vi "main.vi"() -> ()   [LabVIEW 2019]
uses:
  CodeModule/gui/RUNNING.ctl
  CodeModule/gui/LeSSeN.ctl
  CodeModule/gui/add.ctl
  CodeModule/core/core_reportMode.ctl
  CodeModule/core/core_reportCfg.ctl
  CodeModule/gui/ps_setting.ctl
  CodeModule/gui/LIMIT DATA.ctl
  CodeModule/instrument/Instrument.lvclass
  CodeModule/core/core_dataCluster.ctl
panel:
  out "日期/时间":string
  in  "Save data":bool
  in  "Settings":bool
  out "Torque":T1
  out "ECU":T1
  out "Load":T1
  out "DC Power":T1
  out "ECU SATE":i16
  out "System EFF":dbl format="%#_4f"
  out "ECU EFF":dbl format="%#_4f"
  out "Motor":dbl format="%#_5f"
  out "Motor EFF":dbl format="%#_4f"
  out "Motor Power":dbl format="%#_4g"
  out "Pha Power":dbl format="%#_6f"
  out "Pha Current":dbl format="%#_4f"
  out "Pha V":dbl format="%#_4f"
  out "DC Power":dbl format="%#_4f"
  out "Toque":dbl format="%#_4f"
  out "Motor":dbl format="%#_4g"
  out "Drive":dbl format="%#_4f"
  out "Logic V":dbl format="%#_4g"
  out "Temp 2":dbl format="%#_4f"
  out "Temp 1":dbl format="%#_4f"
  out "Speed":dbl format="%#_5f"
  out "Torque":dbl format="%#_4f"
  out "DCCurrent":dbl format="%#_5f"
  out "DC V":dbl format="%#_4f"
  in  "ECU ACK":bool
  in  "load mode":enum32{"torque", "spedd"}(tab)
  in  "Set LoadDivide":dbl(slide) min=0.0 max=2000.0 scale=0.0..5000.0
  in  "Load NM -":T2
  in  "LoadNM+":T3
  out "Load Divide":dbl(knob) scale=1.0..5000.0 scale format="%#_4g"
  in  "StepDivide":dbl
  in  "LOAD ACK Nm":bool
  in  "LOAD ACK":bool
  in  "设定Load[rpm]":i32(slide) min=0 max=4000 step=1 scale=0.0..4000.0
  in  "rpm -":T2
  in  "rpm +":T3
  out "r/m":dbl(knob) scale=0.0..4000.0 scale format="%#.4g"
  in  "Step rpm":i32
  in  "Step Torque":dbl
  out "Troque N/m":dbl(knob) scale=0.0..200.0 scale format="%#_4g"
  in  "Nm -":T2
  in  "Nm +":T3
  in  "Set Torque[Nm]":sgl(slide) min=0 max=200 step=0.1 scale=0.0..200.0
  in  "load direction":bool
  in  "finish":bool
  out "State":string
  out "Finish Time":timestamp format="%<%H:%M:%S\n%x>T"
  out "Start Time":timestamp format="%<%H:%M:%S\n%x>T"
  in  "report cfg":T4
  in  "Duration [min]":i32=30
  in  "Data Mode":T5
  in  "Report File Path":path
  in  "Profile File Path":path
  in  "Cycle Time":i32=1
  out "DATA":string[][](table)
  in  "load torque":bool
  out "CYC  Times":dbl format="%#_7g"
  out "Run Time":dbl format="%<%H:%M:%S>t"
  in  "load 2":bool
  in  "ecu":bool
  in  "ps":bool
  in  "zlg":bool
  in  "play":bool
  in  "emergency stop":bool
  # "BST-1500-22KW电力测功机系统"
  # "MOTOR"
  # "rpm"
  # "N/m"
  # "KW"
  # "DC Power"
  # "V"
  # "A"
  # "KW"
  # "ZLG"
  # "KW"
  # "V"
  # "A"
  # "%"
  # "%"
  # "%"
  # "ECU"
  # "V"
  # "℃"
  # "℃"
  # "ECU"
  # "rpm"
  # "℃"
  # "Temp"
  # "℃"
  # "℃"
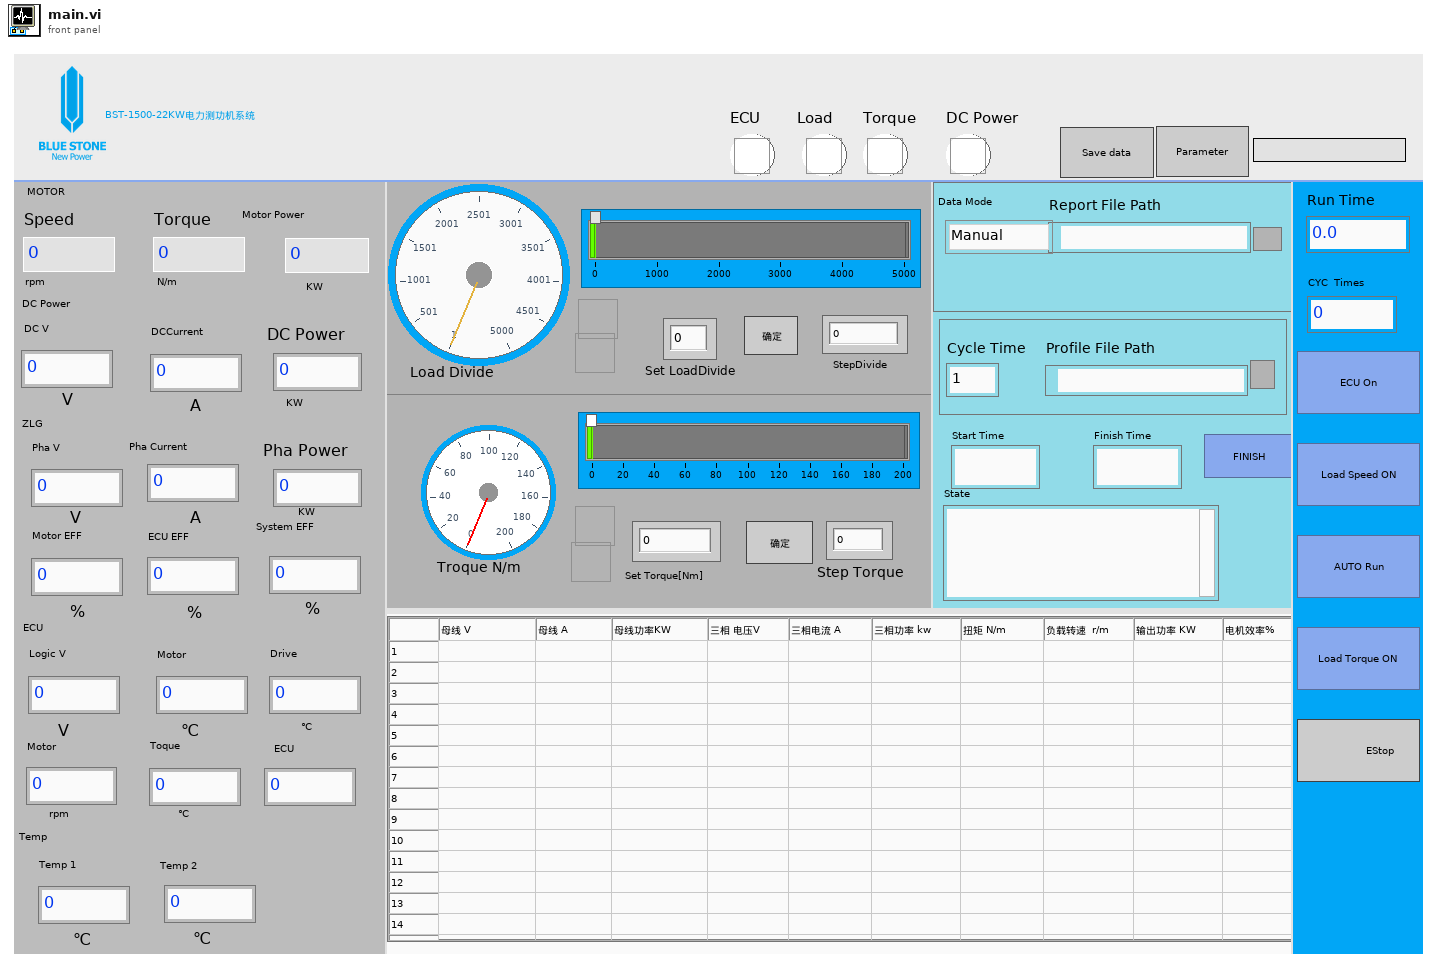
[diagram p1: front panel]
types:
  T1 = typedef "RUNNING.ctl" = bool
  T2 = typedef "LeSSeN.ctl" = bool
  T3 = typedef "add.ctl" = bool
  T4 = typedef "core_reportCfg.ctl" = cluster{"Path":path, "duration(min)":i32, "mode":T5}
  T5 = typedef "core_reportMode.ctl" = enum16{"Manual", "Automatic"}
  T6 = typedef "LIMIT DATA.ctl" = cluster{"Motor Temp Limit ":dbl, " Motor Speed Limit ":dbl, "AXIS Temp Limit  ":dbl, " Torque Limit":dbl, " Speed   limt":dbl}
  T7 = typedef "ps_setting.ctl" = cluster{"母线电压":sgl, "母线电流":sgl, "过载电压":sgl, "过载电流":sgl}
  T8 = typedef "select.ctl" = bool
  T9 = cluster{"Error event ref out":refnum<user-event>, "ecuData":refnum<user-event>}
  T10 = typedef "core_dataRefCluster.ctl" = cluster{"modbus":T11, "ecu":T11, "test":T11}
  T11 = typedef "core_dataRef.ctl" = refnum<queue>
  T12 = typedef "core_dataCluster.ctl" = cluster{"cmd":string, "data":variant}
  T13 = cluster{"母线电压":sgl, "母线电流":sgl, "过载电压":sgl, "过载电流":sgl, "ps":bool}
  T14 = typedef "core_setup.ctl" = cluster{"time":i32, "torque":dbl, "speed":i32}
  T15 = typedef "profile value.ctl" = cluster{"time in":i32, "speed":dbl, "Torque":dbl}
  T16 = typedef "Instrument.lvclass/instr_dataCluster.ctl" = cluster{"电源电压 V":dbl, "电源电流A":dbl, "扭矩N/m":dbl, "速度r/M":dbl, "温度℃":dbl[], "流量计L/M":dbl[]}
  T17 = typedef "core shown data.ctl" = cluster{"SHOWN":dbl[], "temp 2":dbl, "ECU EFF":dbl, "SYS EFF":dbl, "temp 1":dbl}
  T18 = enum8{"Enabled", "Disabled", "Disabled and Grayed Out"}
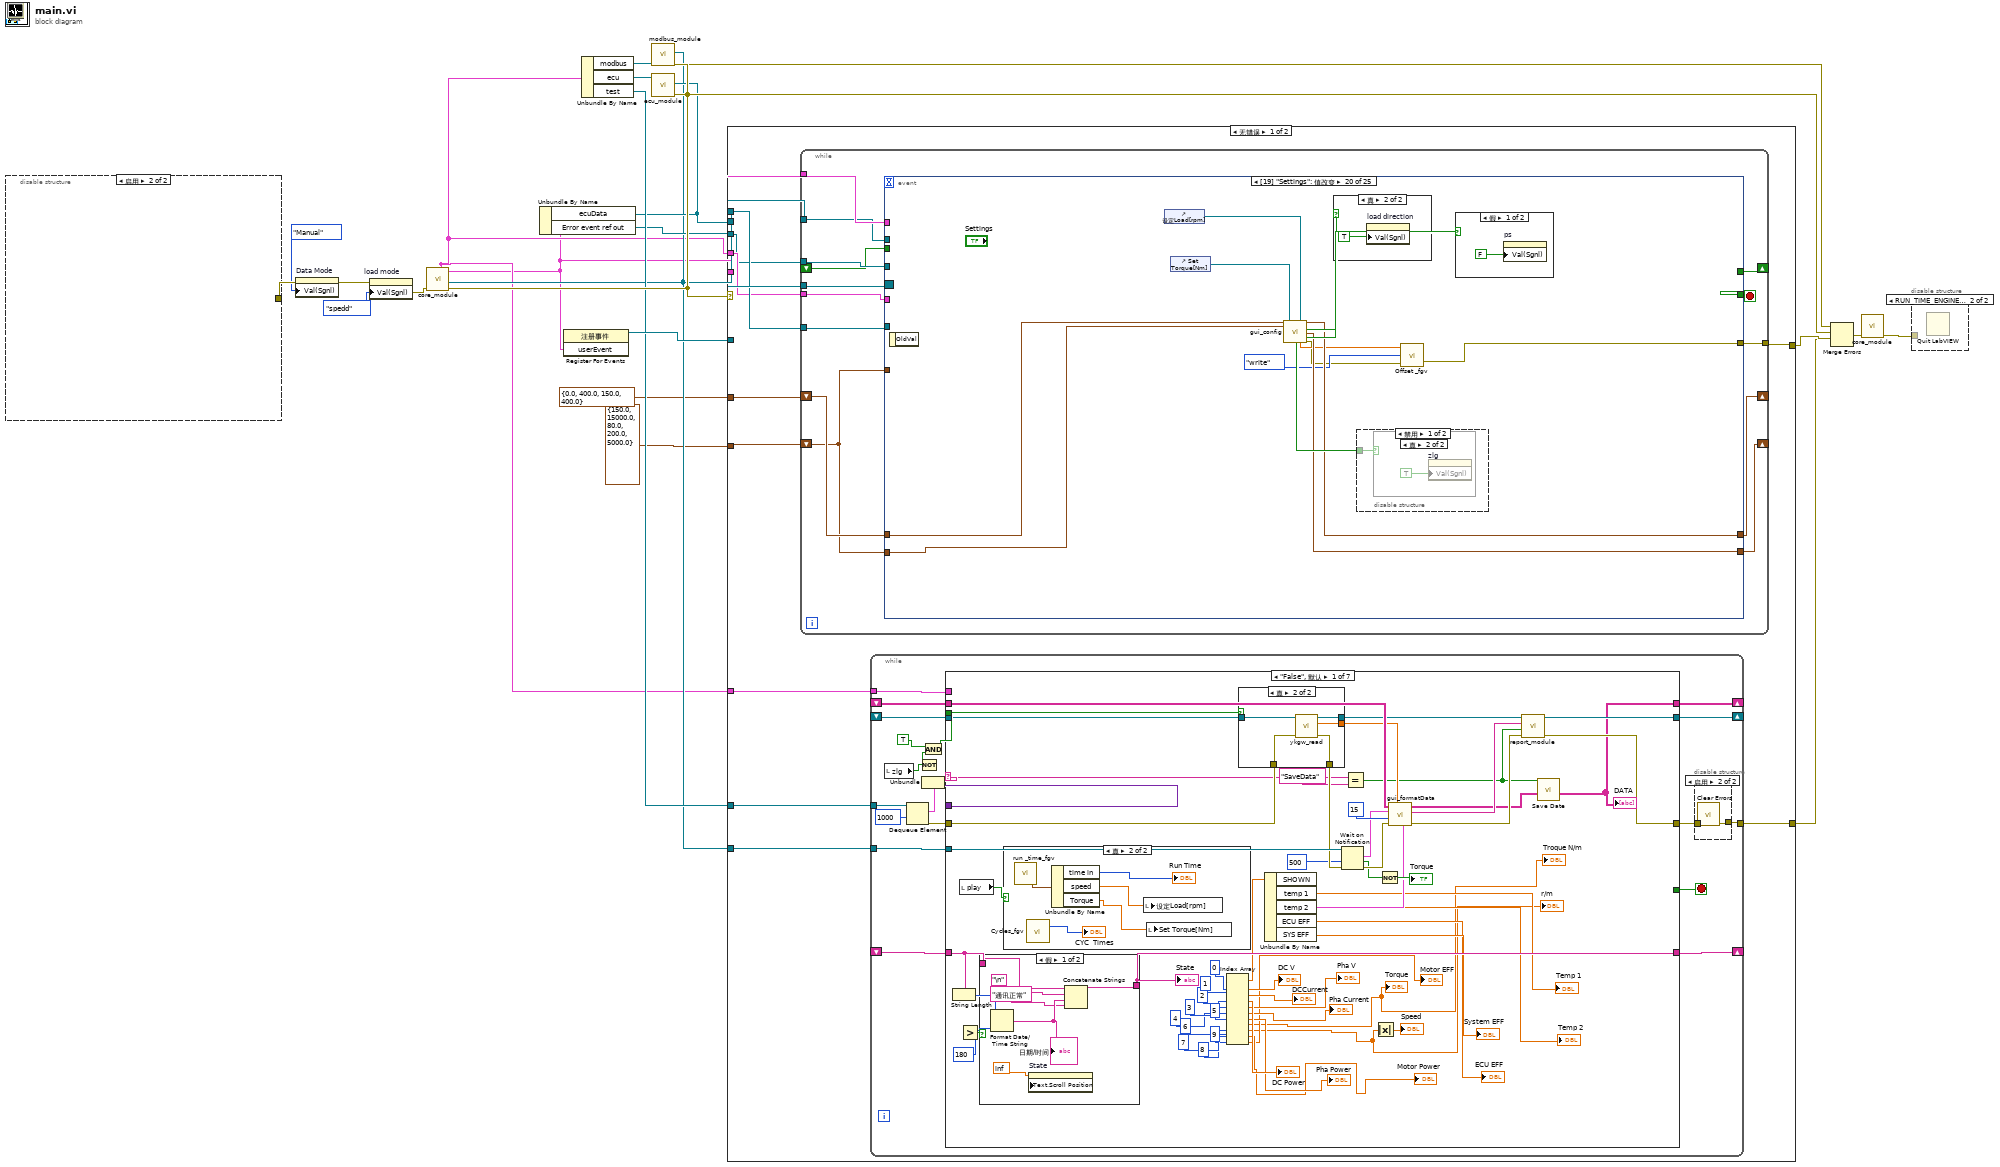
[diagram p0: block diagram]
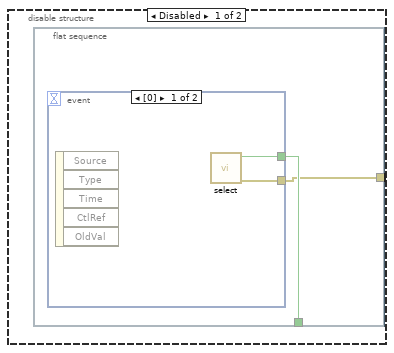
[diagram p2: hidden frame]
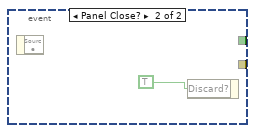
[diagram p3: hidden frame]
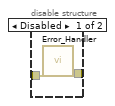
[diagram p4: hidden frame]
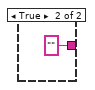
[diagram p5: hidden frame]
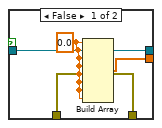
[diagram p6: hidden frame]
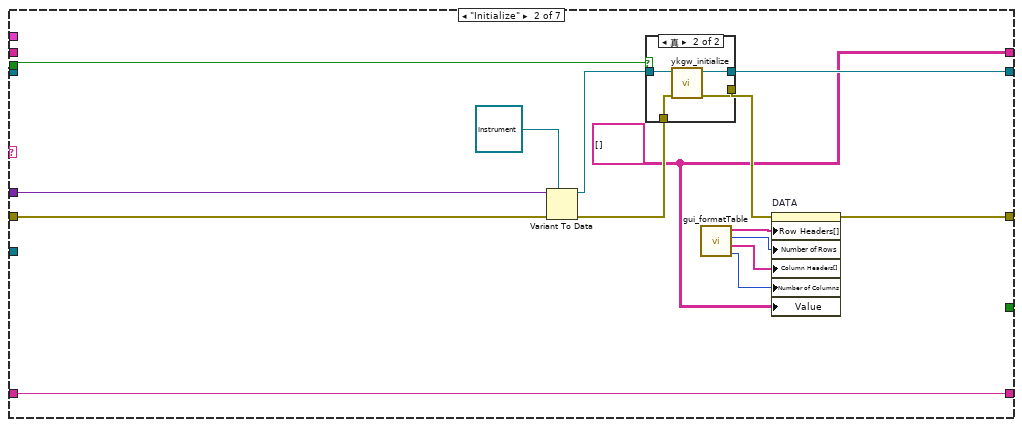
[diagram p8: hidden frame]
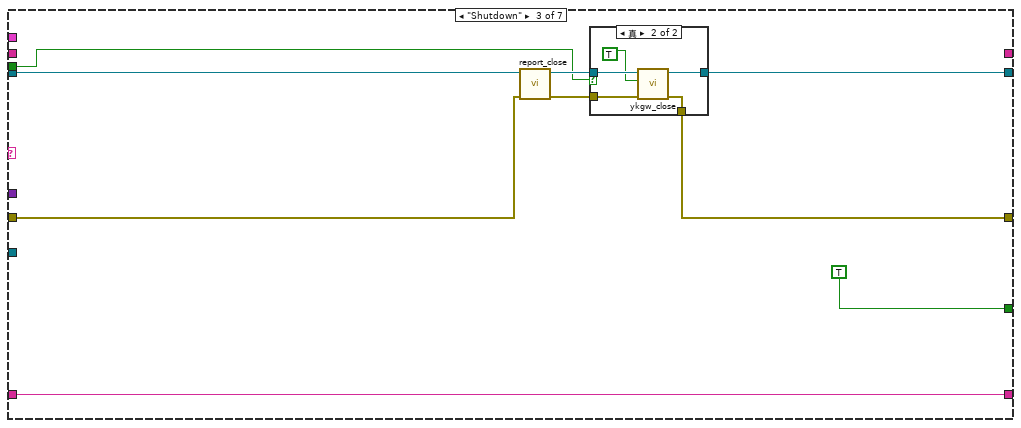
[diagram p10: hidden frame]
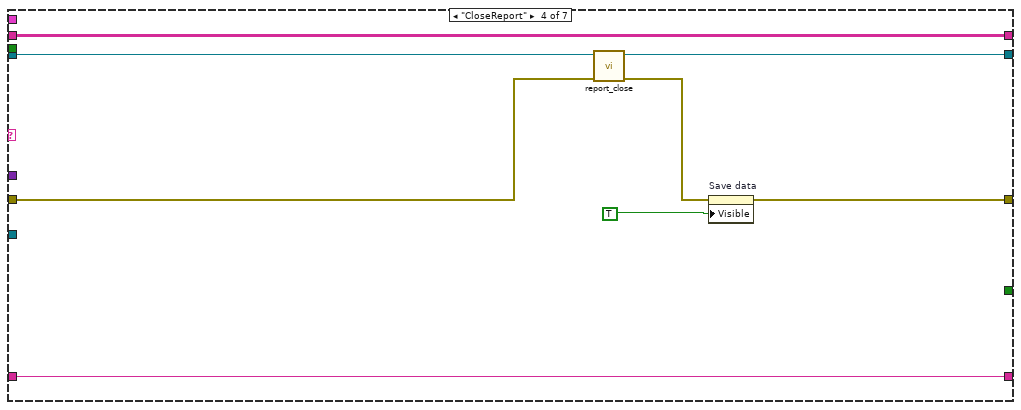
[diagram p12: hidden frame]
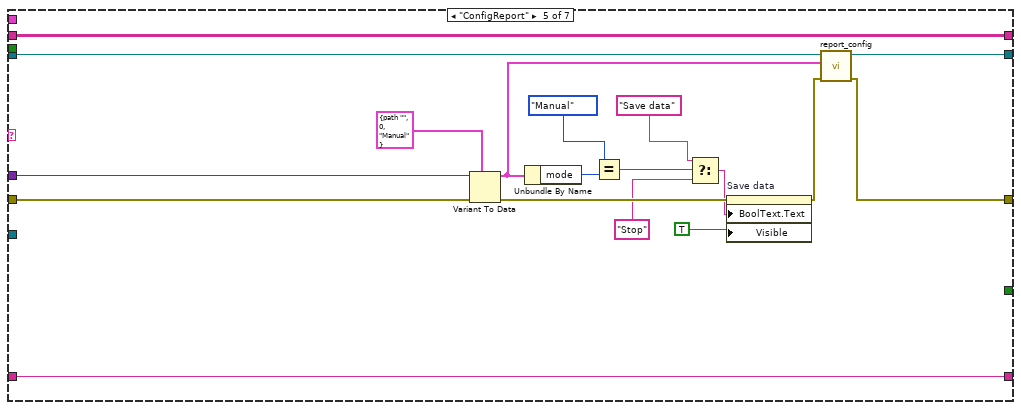
[diagram p13: hidden frame]
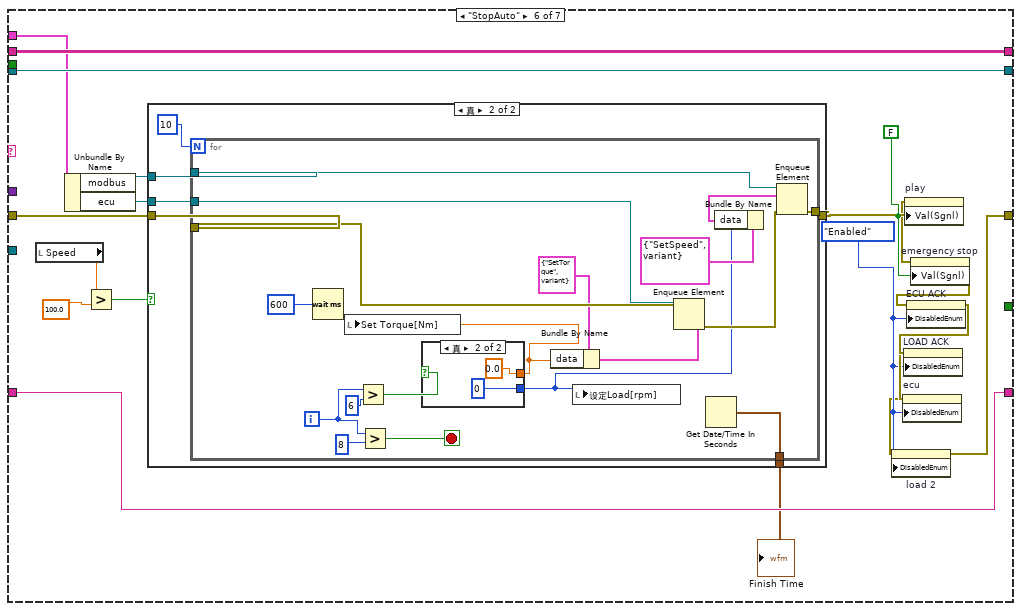
[diagram p14: hidden frame]
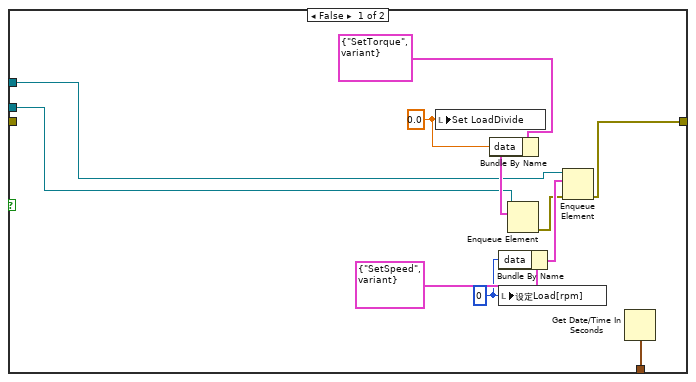
[diagram p15: hidden frame]
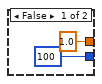
[diagram p16: hidden frame]
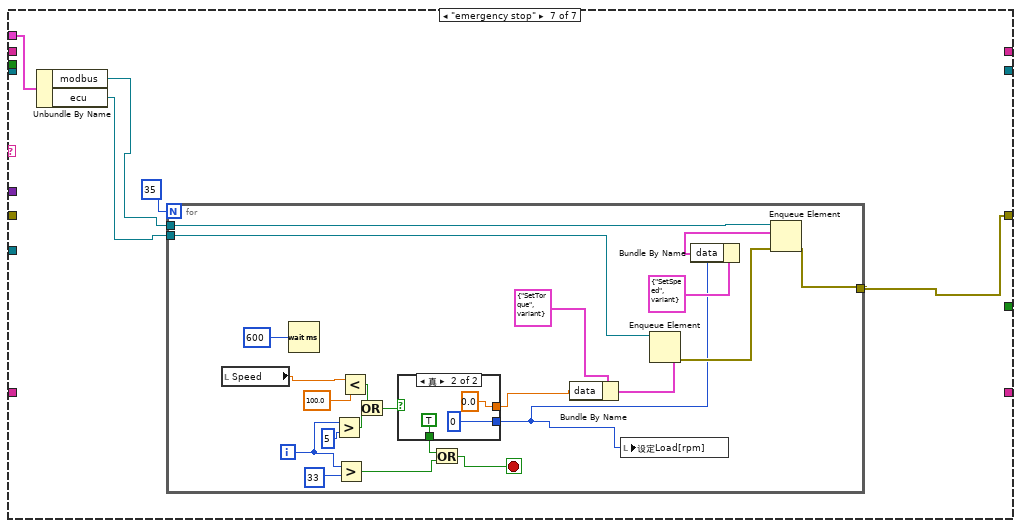
[diagram p17: hidden frame]
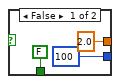
[diagram p18: hidden frame]
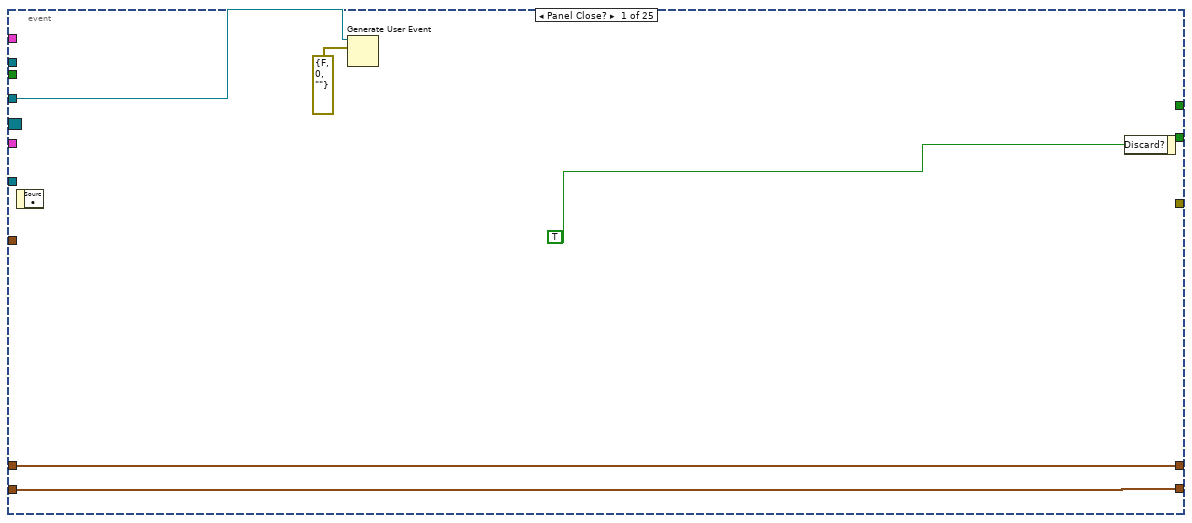
[diagram p19: hidden frame]
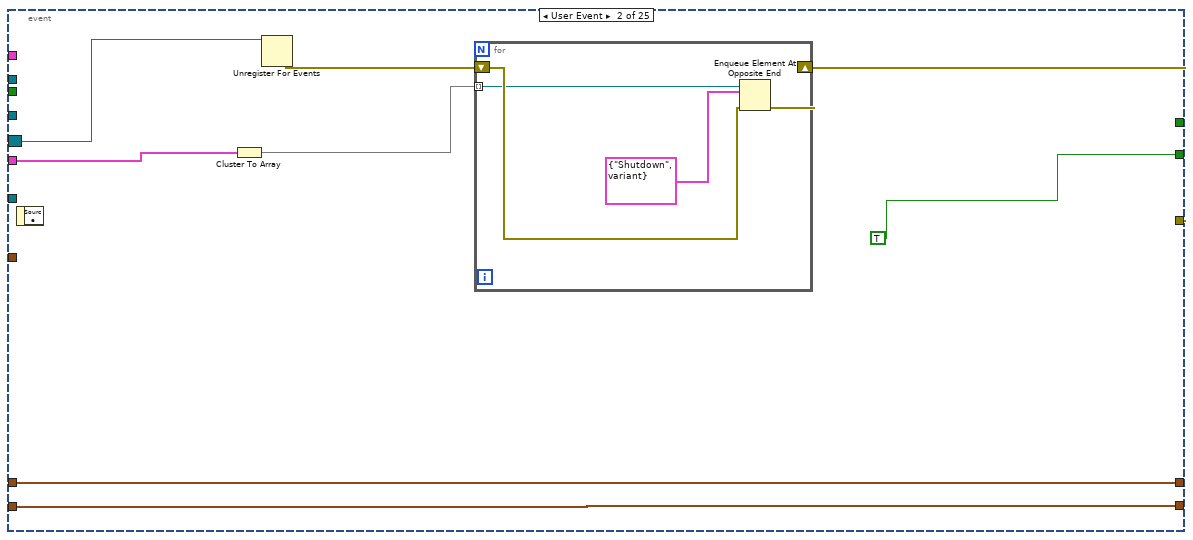
[diagram p20: hidden frame]
diagram:
  n1 = disable-structure shown="启用" {
    disable-tunnel: [w24 _] -> w5
    frame Disabled {
      n2 = flat-sequence {
        tunnel: [w26] -> _
        tunnel: [w25] -> w24
        frame #0 {
          n3 = event shown="[0]" {
            selector: _ -> [_ _]
            dyn-events: _ -> [_ _]
            timeout: _ -> [_ _]
            tunnel: [w28 _] -> w25
            tunnel: [w27 _] -> w26
            event #0 (no event record) {
              n4 = event-data() -> ()  [unwired: 1 in, 5 out]
              n5 = call "select.vi"() -> ("out"=w27:T8, "error out"=w28:errorcluster)  [unwired: 9 in]
            }
            event Panel Close? {
              n6 = event-data() -> ()  [unwired: 1 in, 1 out]
              n7 = event-data("Discard?"=TRUE) -> ()  [unwired: 1 in, 1 out]
            }
          }
        }
      }
    }
    frame Enabled {
    }
  }
  n8 = property on="Data Mode" class="Enum (严格)"(error in=w5, "Val(Sgnl)"=core_reportMode."Manual" ("值(信号)")) -> (error out=w3:errorcluster)  [unwired: 1 in, 1 out]
  n9 = property on="load mode" class="TabCtl (严格)"(error in=w3, "Val(Sgnl)"=enum32{"torque", "spedd"}."spedd" ("load mode")) -> (error out=w1:errorcluster)  [unwired: 1 in, 1 out]
  n10 = call "core_module.vi"("error in (no error)"=w1) -> ("error out"=w19:errorcluster, "modbusData"=w11:refnum<notifier>, "userEvent"=w6:T9, "Cluster"=w9:T10)  [unwired: 6 in, 1 out]
  n11 = Unbundle By Name(w6) -> ("ecuData"=w12:refnum<user-event>, "Error event ref out"=w13:refnum<user-event>)
  n12 = register-events(w6) -> (reference out=w23:refnum<event-registration>)  [unwired: 2 in, 1 out]
  n13 = Unbundle By Name(w9) -> ("modbus"=w16:T11, "ecu"=w15:T11, "test"=w14:T11)
  n14 = call "modbus_module.vi"("error in (no error)"=w19, "User Event"=w11, "queue in"=w16) -> ("error out"=w18:errorcluster)  [unwired: 8 in]
  n15 = call "ecu_module.vi"("error in (no error)"=w19, "ecuData"=w12, "queue in"=w15) -> ("error out"=w20:errorcluster)  [unwired: 8 in]
  n16 = case shown="无错误" w19 {
    tunnel: w6 -> [w42 _]
    tunnel: w23 -> [w41 _]
    tunnel: w9 -> [w31 _]
    tunnel: [w33 _] -> w22
    tunnel: w14 -> [w40 _]
    tunnel: [w39 _] -> w17
    tunnel: w11 -> [w38 _]
    tunnel: w13 -> [w30 _]
    tunnel: w12 -> [w37 _]
    tunnel: w11 -> [w32 _]
    tunnel: T7 {"母线电压"=0.0, "母线电流"=400.0, "过载电压"=150.0, "过载电流"=400.0} ("PS Setting") -> [w34 _]
    tunnel: w9 -> [w36 _]
    tunnel: T6 {"Motor Temp Limit "=150.0, " Motor Speed Limit "=15000.0, "AXIS Temp Limit  "=80.0, " Torque Limit"=200.0, " Speed   limt"=5000.0} ("LIMIT") -> [w35 _]
    frame No Error {
      n17 = while {
        tunnel: w42 -> [w313]
        tunnel: w41 -> [w312]
        tunnel: w30 -> [w311]
        tunnel: w37 -> [w310]
        tunnel: w32 -> [w309]
        shift-right: [w305] -> _
        shift-left: _ -> [w308]
        shift-right: [w302] -> _
        shift-left: w35 -> [w300]
        shift-right: [w303] -> _
        shift-left: w34 -> [w307]
        tunnel: [w304] -> w33
        tunnel: w31 -> [w301]
        stop <- w306 stop-if-true
        n18 = event shown="[19] \"Settings\": 值改变" {
          selector: w312 -> [_ w326 _ _ _ _ _ _ _ _ _ _ _ _ _ _ _ _ _ _ _ _ _ _ _]
          dyn-events: _ -> [_ _ _ _ _ _ _ _ _ _ _ _ _ _ _ _ _ _ _ _ _ _ _ _ _]
          timeout: _ -> [_ _ _ _ _ _ _ _ _ _ _ _ _ _ _ _ _ _ _ _ _ _ _ _ _]
          tunnel: w313 -> [_ _ _ _ _ _ _ _ _ _ _ _ _ _ _ _ _ _ _ _ _ _ _ _ _]
          tunnel: w301 -> [_ w324 _ w378 w394 w415 w423 w428 w446 w477 w491 w508 w531 w542 w557 w580 w596 w607 w612 _ w671 w699 w708 _ w764]
          tunnel: [_ w322 w344 w379 w393 w401 w417 w429 w441 w472 w492 w509 w529 w540 w556 w574 w586 w605 w617 w629 w666 w698 w707 w751 w758] -> w304
          tunnel: w311 -> [w317 _ _ _ _ _ _ _ _ _ _ _ _ _ _ _ _ _ _ _ _ _ _ _ _]
          tunnel: w310 -> [_ _ _ _ _ _ _ _ _ _ _ _ _ _ _ _ _ _ _ _ _ _ _ _ _]
          tunnel: w309 -> [_ _ w361 _ _ _ _ _ _ _ _ _ _ _ _ _ _ _ _ _ _ _ _ _ _]
          tunnel: w308 -> [_ _ w360 _ w390 _ _ _ _ _ _ _ _ _ _ _ _ _ _ _ _ _ _ _ _]
          tunnel: w300 -> [_ _ w343 _ _ _ _ _ _ _ _ _ _ _ _ _ _ _ _ _ _ _ _ _ _]
          tunnel: w300 -> [w314 w319 w340 w375 w389 w402 w416 w424 w440 w461 w487 w503 w524 w536 w553 w575 w585 w600 w616 w634 w656 w683 w704 w749 w754]
          tunnel: w307 -> [w316 w320 w342 w376 w391 w403 w418 w425 w442 w462 w488 w504 w525 w537 w554 w576 w587 w601 w621 w635 w657 w684 w705 w750 w755]
          tunnel: [w314 w319 w340 w375 w389 w402 w416 w424 w440 w461 w487 w503 w524 w536 w553 w575 w585 w600 w616 w632 w656 w683 w704 w749 w754] -> w302
          tunnel: [_ TRUE _ _ _ _ _ _ _ _ _ _ _ _ _ _ _ _ _ _ _ _ _ _ _] -> w306
          tunnel: [_ _ w341 _ w390 _ _ _ _ _ _ _ _ _ _ _ _ _ w615 _ _ _ _ _ _] -> w305
          tunnel: [w316 w320 w342 w376 w391 w403 w418 w425 w442 w462 w488 w504 w525 w537 w554 w576 w587 w601 w621 w633 w657 w684 w705 w750 w755] -> w303
          event Panel Close? {
            n19 = event-data() -> ()  [unwired: 1 in, 1 out]
            n20 = Generate User Event(user event=w317, event data cluster=errorcluster {"status"=FALSE, "code"=0, "source"=""} ("event data")) -> ()  [unwired: 2 in, 2 out]
            n21 = event-data("Discard?"=TRUE) -> ()  [unwired: 1 in, 1 out]
          }
          event User Event {
            n22 = event-data() -> ()  [unwired: 1 in, 1 out]
            n23 = Cluster To Array(cluster=w324) -> (array=w323:T11[])
            n24 = Unregister For Events(event registration refnum=w326) -> (error out=w325:errorcluster)  [unwired: 1 in]
            n25 = for {
              tunnel: w323 -> [w327] mode=indexing
              shift-right: [w328] -> w322
              shift-left: w325 -> [w330]
              n26 = Enqueue Element At Opposite End(queue=w327, element=T12 {"cmd"="Shutdown", "data"=variant}, error in (no error)=w330) -> (error out=w328:errorcluster)  [unwired: 1 in, 2 out]
            }
          }
          event User Event {
            n27 = event-data() -> ("MCU_MotTq"=→"Toque":dbl, "MCU_MotBusU"=→"Logic V":dbl, "MCU_MotSpd"=w331:dbl, "MCU_MotCtrlrT"=→"Drive":dbl, "MCU_MotBodyT"=→"Motor":dbl, "MCU 状态"=w336:bool)  [unwired: 1 in, 2 out]
            "Motor" <- w331
            n28 = Unbundle By Name(w343) -> ("Motor Temp Limit"=w354:dbl, "Motor Speed Limit"=w339:dbl, "AXIS Temp Limit"=w359:dbl, "Torque Limit"=w352:dbl, "Speed   limt"=w351:dbl)
            n29 = local read "Temp 1"() -> (w358:dbl)
            n30 = local read "Torque"() -> (w347:dbl)
            n31 = local read "Speed"() -> (w345:dbl)
            n32 = local read "Motor"() -> (w355:dbl)
            n33 = Greater?(x=w331, y=w339) -> (0:w338:bool)
            n34 = Greater?(x=w358, y=w359) -> (0:w348:bool)
            n35 = Greater?(x=w345, y=w351) -> (0:w350:bool)
            n36 = Absolute Value(x=w347) -> (abs(x)=w346:dbl)
            n37 = Greater?(x=w355, y=w354) -> (0:w356:bool)
            n38 = Greater?(x=w346, y=w352) -> (0:w353:bool)
            n39 = Compound Arithmetic op=OR ("复合运算")(w353, w356, w350, w348, w338) -> (w349:bool)
            n40 = Boolean To (0,1)(Boolean=w336) -> (0, 1=→"ECU SATE":i16)
            n41 = case shown="假" w349 {
              tunnel: [FALSE TRUE] -> w337
              frame False {
              }
              frame True {
              }
            }
            n42 = disable-structure shown="启用" {
              disable-tunnel: w361 -> [w367 _]
              disable-tunnel: w360 -> [w365 _]
              disable-tunnel: [w364 _] -> w344
              disable-tunnel: [w363 _] -> w341
              frame Disabled {
                n43 = call "gui_checkEmergencyStop.vi"("Check"=w365, "modbusData"=w367) -> ("error out"=w366:errorcluster, "Stop"=w362:bool, "Continue check"=w363:bool)  [unwired: 7 in]
                n44 = case shown="真" w362 {
                  tunnel: w366 -> [w368 w372]
                  tunnel: w362 -> [_ w371]
                  tunnel: [w368 w370] -> w364
                  frame False {
                  }
                  frame True {
                    n45 = Not(x=w371) -> (.not. x?=w369:bool)
                    n46 = property on="emergency stop" class="Bool (严格)"(error in=w372, "Val(Sgnl)"=w369) -> (error out=w370:errorcluster)  [unwired: 1 in, 1 out]
                  }
                }
              }
              frame Enabled {
              }
            }
            n47 = property on="emergency stop" class="Bool (严格)"("Val(Sgnl)"=w337) -> ()  [unwired: 2 in, 2 out]
          }
          event "ps": Value Change {
            n48 = event-data() -> ()  [unwired: 1 in, 1 out]
            n49 = Unbundle By Name(w376) -> ("母线电压"=w386:sgl, "母线电流"=w385:sgl, "过载电压"=w384:sgl, "过载电流"=w383:sgl)
            n50 = Bundle(cluster=T13 {"母线电压"=0.0, "母线电流"=0.0, "过载电压"=0.0, "过载电流"=0.0, "ps"=FALSE} ("簇"), "母线电压"=w386, "母线电流"=w385, "过载电压"=w384, "过载电流"=w383, "ps"="ps") -> (w381:T13)
            n51 = Bundle By Name(cluster=T12 {"cmd"="PS", "data"=variant} ("element"), "data"=w381) -> (w387:T12)
            n52 = Unbundle By Name(w378) -> ("modbus"=w377:T11)
            n53 = Enqueue Element(queue=w377, element=w387) -> (error out=w379:errorcluster)  [unwired: 2 in, 2 out]
            "DC Power" <- "ps"
          }
          event "zlg": Value Change {
            n54 = event-data() -> ("NewVal"=w392:bool)  [unwired: 1 in]
            n55 = disable-structure shown="禁用" {
              disable-tunnel: w394 -> [w400 _]
              disable-tunnel: [w398 _] -> w393
              disable-tunnel: w392 -> [w395 _]
              frame Disabled {
                n56 = Unbundle By Name(w400) -> ("modbus"=w399:T11)
                n57 = Bundle By Name(cluster=T12 {"cmd"="EnableChiller", "data"=variant} ("element"), "data"=w395) -> (w396:T12)
                n58 = Enqueue Element(queue=w399, element=w396) -> (error out=w398:errorcluster)  [unwired: 2 in, 2 out]
              }
              frame Enabled {
              }
            }
          }
          event "ecu": Value Change {
            n59 = event-data() -> ("NewVal"=w407:bool)  [unwired: 1 in]
            "ECU" <- w407
            n60 = Unbundle By Name(w415) -> ("ecu"=w414:T11)
            n61 = Not(x=w407) -> (.not. x?=w406:bool)
            n62 = Select(t="LaunchDaemon", s=w407, f="StopDaemon") -> (s? t:f=w411:string)
            n63 = local read "Set Torque[Nm]"() -> (w404:sgl)
            n64 = Bundle By Name(cluster=T12 {"cmd"="", "data"=variant} ("element"), "cmd"=w411, "data"=w404) -> (w409:T12)
            n65 = Enqueue Element(queue=w414, element=w409) -> (error out=w408:errorcluster)  [unwired: 2 in, 2 out]
            n66 = control-ref of="This VI"() -> (w405:refnum<vi>)
            n67 = property class="VI"(reference=w405, error in=w408, "Front Panel.Closeable"=w406) -> (error out=w401:errorcluster)  [unwired: 1 out]
          }
          event "ECU ACK": Value Change {
            n68 = event-data() -> ()  [unwired: 1 in, 1 out]
            n69 = local read "Set Torque[Nm]"() -> (w419:sgl)
            n70 = Bundle By Name(cluster=T12 {"cmd"="SetTorque", "data"=variant} ("element"), "data"=w419) -> (w421:T12)
            n71 = Unbundle By Name(w423) -> ("ecu"=w422:T11)
            n72 = Enqueue Element(queue=w422, element=w421) -> (error out=w417:errorcluster)  [unwired: 2 in, 2 out]
          }
          event Value Change {
            n73 = event-data() -> ()  [unwired: 1 in, 1 out]
            n74 = Unbundle By Name(w428) -> ("ecu"=w432:T11)
            n75 = case shown="真" "Nm +" {
              tunnel: [_ w435] -> w427
              frame False {
              }
              frame True {
                n76 = for {
                  N: 1 -> [_]
                  shift-right: [w437] -> w435
                  shift-left: "Set Torque[Nm]" -> [w439]
                  tunnel: "Step Torque" -> [w438]
                  n77 = Add(x=w438, y=w439) -> (x+y=w437:dbl)
                }
              }
            }
            n78 = local write "Set Torque[Nm]"(w427) -> ()
            n79 = Bundle By Name(cluster=T12 {"cmd"="SetTorque", "data"=variant} ("element"), "data"=w427) -> (w430:T12)
            n80 = Enqueue Element(queue=w432, element=w430) -> (error out=w429:errorcluster)  [unwired: 2 in, 2 out]
          }
          event Value Change {
            n81 = event-data() -> ()  [unwired: 1 in, 1 out]
            n82 = local read "Set Torque[Nm]"() -> (w445:sgl)
            n83 = Unbundle By Name(w446) -> ("ecu"=w449:T11)
            n84 = case shown="真" "Nm -" {
              tunnel: w445 -> [_ w451]
              tunnel: [_ w452] -> w444
              frame False {
              }
              frame True {
                n85 = Greater Than 0?(x=w451) -> (x > 0?=w450:bool)
                n86 = case shown="真" w450 {
                  tunnel: [0.0 w456] -> w452
                  tunnel: w451 -> [_ w454]
                  frame False {
                  }
                  frame True {
                    n87 = local read "Step Torque"() -> (w455:dbl)
                    n88 = for {
                      N: 1 -> [_]
                      shift-right: [w459] -> w456
                      shift-left: w454 -> [w460]
                      tunnel: w455 -> [w458]
                      n89 = Subtract(x=w460, y=w458) -> (x-y=w459:dbl)
                    }
                  }
                }
              }
            }
            n90 = local write "Set Torque[Nm]"(w444) -> ()
            n91 = Bundle By Name(cluster=T12 {"cmd"="SetTorque", "data"=variant} ("element"), "data"=w444) -> (w447:T12)
            n92 = Enqueue Element(queue=w449, element=w447) -> (error out=w441:errorcluster)  [unwired: 2 in, 2 out]
          }
          event "load 2": Value Change {
            n93 = event-data() -> ("NewVal"=w470:bool)  [unwired: 1 in]
            "Load" <- w470
            n94 = Unbundle By Name(w477) -> ("modbus"=w476:T11)
            n95 = Select(t=i16 1, s="load direction", f=i16 2) -> (s? t:f=w468:i16)
            n96 = Select(t=w468, s=w470, f=i16 0) -> (s? t:f=w467:i16)
            n97 = Bundle By Name(cluster=T12 {"cmd"="StartLoad", "data"=variant} ("element"), "data"=w467) -> (w471:T12)
            n98 = local read "设定Load[rpm]"() -> (w464:i32)
            n99 = Enqueue Element(queue=w476, element=w471) -> (queue out=w474:T11, error out=w473:errorcluster)  [unwired: 2 in, 1 out]
            n100 = case shown="真" w470 {
              tunnel: w474 -> [_ w486]
              tunnel: w473 -> [w479 w485]
              tunnel: [w479 w484] -> w472
              tunnel: w471 -> [_ w483]
              tunnel: w464 -> [_ w482]
              frame False {
                n101 = local write "设定Load[rpm]"(0 ("Load Speed [rpm]")) -> ()
              }
              frame True {
                n102 = Bundle By Name(cluster=w483, "cmd"="SetSpeed", "data"=w482) -> (w481:T12)
                n103 = Enqueue Element(queue=w486, element=w481, error in (no error)=w485) -> (error out=w484:errorcluster)  [unwired: 1 in, 2 out]
              }
            }
          }
          event Value Change {
            n104 = event-data() -> ()  [unwired: 1 in, 1 out]
            n105 = Unbundle By Name(w491) -> ("modbus"=w495:T11)
            n106 = case shown="真" "rpm +" {
              tunnel: [_ w497] -> w489
              frame False {
              }
              frame True {
                n107 = for {
                  N: 1 -> [_]
                  shift-right: [w500] -> w497
                  shift-left: "设定Load[rpm]" -> [w502]
                  tunnel: "Step rpm" -> [w501]
                  n108 = Add(x=w501, y=w502) -> (x+y=w500:i32)
                }
              }
            }
            n109 = local write "设定Load[rpm]"(w489) -> ()
            n110 = Bundle By Name(cluster=T12 {"cmd"="SetSpeed", "data"=variant} ("element"), "data"=w489) -> (w493:T12)
            n111 = Enqueue Element(queue=w495, element=w493) -> (error out=w492:errorcluster)  [unwired: 2 in, 2 out]
          }
          event Value Change {
            n112 = event-data() -> ()  [unwired: 1 in, 1 out]
            n113 = Unbundle By Name(w508) -> ("modbus"=w512:T11)
            n114 = local read "设定Load[rpm]"() -> (w506:i32)
            n115 = case shown="真" "rpm -" {
              tunnel: w506 -> [_ w514]
              tunnel: [_ w515] -> w507
              frame False {
              }
              frame True {
                n116 = Greater Than 0?(x=w514) -> (x > 0?=w513:bool)
                n117 = case shown="真" w513 {
                  tunnel: w514 -> [_ w519]
                  tunnel: [0 w518] -> w515
                  frame False {
                  }
                  frame True {
                    n118 = property on="Step rpm" class="DigNum (严格)"() -> ("Value"=w517:i32)  [unwired: 2 in, 2 out]
                    n119 = for {
                      N: 1 -> [_]
                      tunnel: w517 -> [w522]
                      shift-right: [w521] -> w518
                      shift-left: w519 -> [w523]
                      n120 = Subtract(x=w523, y=w522) -> (x-y=w521:i32)
                    }
                  }
                }
              }
            }
            n121 = local write "设定Load[rpm]"(w507) -> ()
            n122 = Bundle By Name(cluster=T12 {"cmd"="SetSpeed", "data"=variant} ("element"), "data"=w507) -> (w510:T12)
            n123 = Enqueue Element(queue=w512, element=w510) -> (error out=w509:errorcluster)  [unwired: 2 in, 2 out]
          }
          event "LOAD ACK Nm": Value Change {
            n124 = event-data() -> ()  [unwired: 1 in, 1 out]
            n125 = Unbundle By Name(w531) -> ("modbus"=w530:T11)
            n126 = local read "Set LoadDivide"() -> (w526:dbl)
            n127 = case shown="真" "LOAD ACK Nm" {
              tunnel: w526 -> [_ w534]
              tunnel: [_ w533] -> w528
              frame False {
              }
              frame True {
                n128 = To Double Precision Float(number=w534) -> (double precision float=w532:dbl)
                n129 = local write "Load Divide"(w532) -> ()
                n130 = Bundle By Name(cluster=T12 {"cmd"="SetLoadTorque", "data"=variant} ("element"), "data"=w532) -> (w533:T12)
              }
            }
            n131 = Enqueue Element(queue=w530, element=w528) -> (error out=w529:errorcluster)  [unwired: 2 in, 2 out]
          }
          event Value Change {
            n132 = event-data() -> ()  [unwired: 1 in, 1 out]
            n133 = Unbundle By Name(w542) -> ("modbus"=w544:T11)
            n134 = case shown="真" "LoadNM+" {
              tunnel: [_ w547] -> w539
              frame False {
              }
              frame True {
                n135 = local read "Set LoadDivide"() -> (w545:dbl)
                n136 = for {
                  N: 1 -> [_]
                  shift-right: [w549] -> w547
                  shift-left: "StepDivide" -> [w551]
                  tunnel: w545 -> [w550]
                  n137 = Add(x=w550, y=w551) -> (x+y=w549:dbl)
                }
              }
            }
            "Load Divide" <- w539
            n138 = local write "Set LoadDivide"(w539) -> ()
            n139 = Bundle By Name(cluster=T12 {"cmd"="SetLoadTorque", "data"=variant} ("element"), "data"=w539) -> (w543:T12)
            n140 = Enqueue Element(queue=w544, element=w543) -> (error out=w540:errorcluster)  [unwired: 2 in, 2 out]
          }
          event Value Change {
            n141 = event-data() -> ()  [unwired: 1 in, 1 out]
            n142 = Unbundle By Name(w557) -> ("modbus"=w560:T11)
            n143 = case shown="真" "Load NM -" {
              tunnel: [_ w563] -> w552
              frame False {
              }
              frame True {
                n144 = local read "Set LoadDivide"() -> (w561:dbl)
                n145 = Greater Than 0?(x=w561) -> (x > 0?=w562:bool)
                n146 = case shown="真" w562 {
                  tunnel: w561 -> [_ w567]
                  tunnel: [0.0 w566] -> w563
                  frame False {
                  }
                  frame True {
                    n147 = local read "StepDivide"() -> (w565:dbl)
                    n148 = for {
                      N: 1 -> [_]
                      shift-right: [w570] -> w566
                      shift-left: w567 -> [w571]
                      tunnel: w565 -> [w569]
                      n149 = Subtract(x=w571, y=w569) -> (x-y=w570:dbl)
                    }
                  }
                }
              }
            }
            n150 = local write "Load Divide"(w552) -> ()
            n151 = local write "Set LoadDivide"(w552) -> ()
            n152 = Bundle By Name(cluster=T12 {"cmd"="SetLoadTorque", "data"=variant} ("element"), "data"=w552) -> (w559:T12)
            n153 = Enqueue Element(queue=w560, element=w559) -> (error out=w556:errorcluster)  [unwired: 2 in, 2 out]
          }
          event "load torque": Value Change {
            n154 = event-data() -> ("NewVal"=w572:bool)  [unwired: 1 in]
            n155 = Unbundle By Name(w580) -> ("modbus"=w579:T11)
            n156 = control-ref of="load mode"() -> (w573:refnum<vi>)
            n157 = case shown="假" w572 {
              tunnel: w573 -> [w581 w584]
              frame False {
                n158 = property class="TabCtl (严格)"(reference=w581, "Val(Sgnl)"=enum32{"torque", "spedd"}."spedd" ("值(信号)")) -> ()  [unwired: 1 in, 2 out]
              }
              frame True {
                n159 = property class="TabCtl (严格)"(reference=w584, "Val(Sgnl)"=enum32{"torque", "spedd"}."torque" ("值(信号)")) -> ()  [unwired: 1 in, 2 out]
              }
            }
            n160 = Bundle By Name(cluster=T12 {"cmd"="StartLoadTorqueMode", "data"=variant} ("element"), "data"=w572) -> (w577:T12)
            n161 = Enqueue Element(queue=w579, element=w577) -> (error out=w574:errorcluster)  [unwired: 2 in, 2 out]
          }
          event "load direction": Value Change {
            n162 = event-data() -> ("NewVal"=w594:bool)  [unwired: 1 in]
            n163 = Unbundle By Name(w596) -> ("modbus"=w595:T11)
            n164 = Select(t=i16 1, s=w594, f=i16 2) -> (s? t:f=w590:i16)
            n165 = Bundle By Name(cluster=T12 {"cmd"="StartLoad", "data"=variant} ("element"), "data"=w590) -> (w589:T12)
            n166 = case shown="真" "load 2" {
              tunnel: w595 -> [_ w599]
              tunnel: [_ w598] -> w586
              tunnel: w589 -> [_ w597]
              frame False {
              }
              frame True {
                n167 = Enqueue Element(queue=w599, element=w597) -> (error out=w598:errorcluster)  [unwired: 2 in, 2 out]
              }
            }
          }
          event "LOAD ACK": Value Change {
            n168 = event-data() -> ()  [unwired: 1 in, 1 out]
            n169 = local read "设定Load[rpm]"() -> (w602:i32)
            n170 = Unbundle By Name(w607) -> ("modbus"=w606:T11)
            n171 = case shown="真" "LOAD ACK" {
              tunnel: [_ w609] -> w604
              tunnel: w602 -> [_ w608]
              frame False {
              }
              frame True {
                n172 = Bundle By Name(cluster=T12 {"cmd"="SetSpeed", "data"=variant} ("element"), "data"=w608) -> (w609:T12)
              }
            }
            n173 = Enqueue Element(queue=w606, element=w604) -> (error out=w605:errorcluster)  [unwired: 2 in, 2 out]
          }
          event "emergency stop": Value Change {
            n174 = event-data() -> ()  [unwired: 1 in, 1 out]
            n175 = local read "play"() -> (w620:bool)
            n176 = local read "ECU"() -> (w615:T1)
            n177 = Unbundle By Name(w612) -> ("test"=w611:T11)
            n178 = Not(x=w620) -> (.not. x?=w619:bool)
            n179 = And(x=w615, y="emergency stop") -> (x .and. y?=w613:T1)
            n180 = And(x=w613, y=w619) -> (x .and. y?=w618:T1)
            n181 = case shown="假" w618 {
              tunnel: [_ w622] -> w617
              tunnel: w611 -> [_ w627]
              frame False {
              }
              frame True {
                n182 = Enqueue Element(queue=w627, element=T12 {"cmd"="emergency stop", "data"=variant} ("元素")) -> (error out=w623:errorcluster)  [unwired: 2 in, 2 out]
                n183 = call "estop_fgv.vi"("error in (no error)"=w623, "Boolean"=TRUE, "Enum"=enum16{"set", "get"}."set") -> ("error out"=w622:errorcluster)  [unwired: 7 in, 1 out]
              }
            }
          }
          event "Settings": Value Change {
            n184 = event-data() -> ()  [unwired: 1 in, 1 out]
            n185 = control-ref of="设定Load[rpm]"() -> (w640:refnum<vi>)
            n186 = control-ref of="Set Torque[Nm]"() -> (w639:refnum<vi>)
            n187 = call "gui_config.vi"("PS Setting"=w635, "LIMIT"=w634, "Torque"=w639, "Speed"=w640) -> ("Water mode"=w637:bool, "Offset out"=w631:dbl, "PS Setting out"=w633:T7, "mode out"=w636:bool, "LIMIT  out"=w632:T6, "power mode"=w638:bool, "error out"=w628:errorcluster)  [unwired: 8 in, 1 out]
            n188 = case shown="真" w636 {
              frame False {
                n189 = property on="load direction" class="Bool (严格)"("Val(Sgnl)"=FALSE) -> ()  [unwired: 2 in, 2 out]
              }
              frame True {
                n190 = property on="load direction" class="Bool (严格)"("Val(Sgnl)"=TRUE) -> ()  [unwired: 2 in, 2 out]
              }
            }
            n191 = disable-structure shown="禁用" {
              disable-tunnel: w637 -> [w641 _]
              frame Disabled {
                n192 = case shown="真" w641 {
                  frame False {
                    n193 = property on="zlg" class="Bool (严格)"("Val(Sgnl)"=FALSE) -> ()  [unwired: 2 in, 2 out]
                  }
                  frame True {
                    n194 = property on="zlg" class="Bool (严格)"("Val(Sgnl)"=TRUE) -> ()  [unwired: 2 in, 2 out]
                  }
                }
              }
              frame Enabled {
              }
            }
            n195 = call "Offset _fgv.vi"("error in (no error)"=w628, "mode"=enum16{"read", "write"}."write", "Value  in"=w631) -> ("error out"=w629:errorcluster)  [unwired: 1 out]
            n196 = case shown="假" w638 {
              frame False {
                n197 = property on="ps" class="Bool (严格)"("Val(Sgnl)"=FALSE) -> ()  [unwired: 2 in, 2 out]
              }
              frame True {
                n198 = property on="ps" class="Bool (严格)"("Val(Sgnl)"=TRUE) -> ()  [unwired: 2 in, 2 out]
              }
            }
          }
          event Value Change {
            n199 = event-data() -> ("NewVal"=w654:T5)  [unwired: 1 in]
            n200 = Empty String/Path?(string/path="Report File Path") -> (empty?=w662:bool)
            n201 = Unbundle By Name(w671) -> ("test"=w670:T11)
            n202 = case shown="真" w662 {
              tunnel: [w673 w678] -> w661
              tunnel: "Report File Path" -> [w673 _]
              frame False {
              }
              frame True {
                w674 = path "d:/report" ("基路径")
                n203 = call <vilib>:"Check if File or Folder Exists.vi"("path"=w674) -> ("file or folder exists?"=w676:bool)  [unwired: 8 in, 2 out]
                n204 = Format Date/Time String(time format string (%c)="%Y_%m_%d_%H_%M_%S.csv") -> (date/time string=w679:string)  [unwired: 2 in]
                n205 = case shown="真" w676 {
                  tunnel: [w681 w682] -> w675
                  tunnel: w674 -> [w680 w682]
                  frame False {
                    n206 = Create Folder(path (use dialog)=w680) -> (created path=w681:path)  [unwired: 2 in, 2 out]
                  }
                  frame True {
                  }
                }
                n207 = Build Path(base path=w675, name or relative path=w679) -> (appended path=w678:path)
              }
            }
            n208 = Equal?(x=core_reportMode."Automatic" ("y"), y=w654) -> (x = y?=w651:bool)
            n209 = Equal?(x=core_reportMode."Manual" ("y"), y=w654) -> (x = y?=w650:bool)
            n210 = property on="Save data" class="Bool"("Visible"=w650) -> (error out=w652:errorcluster)  [unwired: 2 in, 1 out]
            n211 = call "report_generateHeader.vi"("error in (no error)"=w652, "Path in"=w661) -> ("error out"=w663:errorcluster, "Path out"=w659:path)  [unwired: 8 in]
            n212 = Not(x=w650) -> (.not. x?=w649:bool)
            n213 = And(x=w649, y=w651) -> (x .and. y?=w648:bool)
            n214 = property on="Duration [min]" class="DigNum (严格)"(error in=w663, "Visible"=w648) -> (error out=w667:errorcluster)  [unwired: 1 in, 1 out]
            n215 = Bundle By Name(cluster="report cfg", "Path"=w659, "mode"="Data Mode", "duration(min)"="Duration [min]") -> (w658:T4)
            n216 = Bundle By Name(cluster=T12 {"cmd"="ConfigReport", "data"=variant} ("Cluster"), "data"=w658) -> (w668:T12)
            n217 = Enqueue Element(queue=w670, element=w668, error in (no error)=w667) -> (error out=w666:errorcluster)  [unwired: 1 in, 2 out]
          }
          event "Report File Path": Value Change {
            n218 = event-data() -> ()  [unwired: 1 in, 1 out]
            n219 = local read "Report File Path"() -> (w694:path)
            n220 = Unbundle By Name(w699) -> ("test"=w691:T11)
            n221 = local read "Duration [min]"() -> (w692:i32)
            n222 = local read "Data Mode"() -> (w693:T5)
            n223 = local read "report cfg"() -> (w697:T4)
            n224 = call "report_generateHeader.vi"("Path in"=w694) -> ("error out"=w689:errorcluster, "Path out"=w685:path)  [unwired: 9 in]
            n225 = Bundle By Name(cluster=w697, "Path"=w685, "mode"=w693, "duration(min)"=w692) -> (w695:T4)
            n226 = Empty String/Path?(string/path=w685) -> (empty?=w687:bool)
            n227 = Bundle By Name(cluster=T12 {"cmd"="ConfigReport", "data"=variant} ("Cluster"), "data"=w695) -> (w690:T12)
            n228 = Not(x=w687) -> (.not. x?=w686:bool)
            n229 = case shown="假" w686 {
              tunnel: ["" w703] -> w688
              frame False {
              }
              frame True {
                n230 = Format Date/Time String() -> (date/time string=w702:string)  [unwired: 3 in]
                n231 = Concatenate Strings(w702, "设置文件保存") -> (w703:string)
              }
            }
            n232 = local write "State"(w688) -> ()
            n233 = Enqueue Element(queue=w691, element=w690, error in (no error)=w689) -> (error out=w698:errorcluster)  [unwired: 1 in, 2 out]
          }
          event "play": Value Change {
            n234 = event-data() -> ()  [unwired: 1 in, 1 out]
            n235 = case shown="真" "play" {
              tunnel: w708 -> [_ w726]
              tunnel: [_ w725] -> w707
              frame False {
              }
              frame True {
                w713 = 2
                n236 = Get Date/Time In Seconds() -> (seconds since 1Jan1904=→"Start Time":timestamp)
                n237 = disable-structure shown="启用" {
                  disable-tunnel: [w734 _] -> w712
                  disable-tunnel: [w733 w737] -> w711
                  disable-tunnel: "Profile File Path" -> [w732 w738]
                  frame Disabled {
                    n238 = call "Data - relative_file_path_handling.vi"("path in"=w732) -> ("error out"=w734:errorcluster, "path out"=w733:path)  [unwired: 9 in]
                  }
                  frame Enabled {
                    n239 = Strip Path(path=w738) -> (stripped path=w736:path, name=w735:string)
                    n240 = Build Path(base path=w736, name or relative path=w735) -> (appended path=w737:path)
                  }
                }
                n241 = call "estop_fgv.vi"("error in (no error)"=w712, "Boolean"=FALSE) -> ("error out"=w722:errorcluster)  [unwired: 8 in, 1 out]
                n242 = call <vilib>:"Check if File or Folder Exists.vi"("error in (no error)"=w722, "path"=w711) -> ("error out"=w715:errorcluster, "file or folder exists?"=w724:bool, "dup path"=w728:path)  [unwired: 7 in]
                n243 = local read "Torque"() -> (w729:T1)
                n244 = Greater Than 0?(x="Cycle Time") -> (x > 0?=w723:bool)
                n245 = property on="ECU ACK" class="Bool"(error in=w715, "DisabledEnum"=w713) -> (error out=w718:errorcluster)  [unwired: 1 in, 1 out]
                n246 = local read "DC Power"() -> (w709:T1)
                n247 = property on="LOAD ACK" class="Bool"(error in=w718, "DisabledEnum"=w713) -> (error out=w717:errorcluster)  [unwired: 1 in, 1 out]
                n248 = local read "Load"() -> (w730:T1)
                n249 = local read "ECU"() -> (w731:T1)
                n250 = property on="ecu" class="Bool (严格)"(error in=w717, "DisabledEnum"=w713) -> (error out=w716:errorcluster)  [unwired: 1 in, 1 out]
                n251 = property on="load 2" class="Bool (严格)"(error in=w716, "DisabledEnum"=w713) -> (error out=w714:errorcluster)  [unwired: 1 in, 1 out]
                n252 = Compound Arithmetic op=AND(w724, w723, w731, w730, w709, w729) -> (w727:T1)
                n253 = case shown="真" w727 {
                  tunnel: w714 -> [w740 w748]
                  tunnel: w728 -> [_ w747]
                  tunnel: w726 -> [_ w744]
                  tunnel: [w741 w743] -> w725
                  tunnel: "Cycle Time" -> [_ w742]
                  frame False {
                    n254 = call "profile_status.vi"("error in (no error)"=w740, "status"=FALSE) -> ("error out"=w741:errorcluster)  [unwired: 9 in]
                  }
                  frame True {
                    n255 = call "load_profile.vi"("error in (no error)"=w748, "Path"=w747) -> ("error out"=w746:errorcluster, "Array"=w745:T14[])  [unwired: 8 in]
                    n256 = call "launch_dynamic_vi.vi"("queue"=w744, "error in (no error)"=w746, "cycle"=w742, "profile"=w745) -> ("error out"=w743:errorcluster)  [unwired: 7 in]
                  }
                }
              }
            }
          }
          event "finish": Value Change {
            n257 = event-data() -> ()  [unwired: 1 in, 1 out]
            n258 = call "estop_fgv.vi"("Boolean"=TRUE, "Enum"=enum16{"set", "get"}."set") -> ("error out"=w751:errorcluster)  [unwired: 8 in, 1 out]
          }
          event "Save data": Value Change {
            n259 = event-data() -> ("CtlRef"=w762:refnum<vi>)  [unwired: 1 in]
            n260 = Unbundle By Name(w764) -> ("test"=w763:T11)
            n261 = property class="Bool"(reference=w762) -> (reference out=w756:refnum<vi>, error out=w757:errorcluster, "BoolText.Text"=w761:string)  [unwired: 1 in]
            n262 = case shown="\"Stop\"" w761 {
              tunnel: [T12 {"cmd"="SaveData", "data"=variant} ("element") T12 {"cmd"="CloseReport", "data"=variant} ("element")] -> w760
              frame "Save data", Default {
              }
              frame "Stop" {
              }
            }
            n263 = Enqueue Element(queue=w763, element=w760, error in (no error)=w757) -> (error out=w759:errorcluster)  [unwired: 1 in, 2 out]
            n264 = Close Reference(reference=w756, error in (no error)=w759) -> (error out=w758:errorcluster)
          }
        }
      }
      n265 = while {
        tunnel: w40 -> [w63]
        shift-right: [w58] -> _
        shift-left: _ -> [w51]
        tunnel: [w57] -> w39
        tunnel: w38 -> [w55]
        shift-right: [w54] -> _
        shift-left: _ -> [w53]
        tunnel: w36 -> [w52]
        shift-right: [w50] -> _
        shift-left: _ -> [w49]
        stop <- w48 stop-if-true
        n266 = local read "zlg"() -> (w47:bool)
        n267 = Dequeue Element(queue=w63, timeout in ms (-1)=1000) -> (element=w62:T12, error out=w60:errorcluster)  [unwired: 1 in, 2 out]
        n268 = Not(x=w47) -> (.not. x?=w46:bool)
        n269 = Unbundle(w62) -> ("cmd"=w61:string, "data"=w59:variant)
        n270 = And(x=TRUE, y=w46) -> (x .and. y?=w44:bool)
        n271 = case shown="\"False\", 默认" w61 {
          selector: w61 -> [w75 _ _ _ _ _ _]
          tunnel: w60 -> [w123 w159 w171 w189 w206 w222 _]
          tunnel: w59 -> [_ w158 _ _ w205 _ _]
          tunnel: [w107 w155 w174 w188 w203 w226 _] -> w58
          tunnel: [w106 w152 w173 w185 w202 w208 w267] -> w43
          tunnel: w55 -> [w122 _ _ _ _ _ _]
          tunnel: [w103 w147 _ w187 w207 w227 _] -> w54
          tunnel: w53 -> [w119 _ _ w187 w207 w227 _]
          tunnel: w52 -> [_ _ _ _ _ w225 w271]
          tunnel: w51 -> [w111 _ w169 w183 w191 w226 _]
          tunnel: [w105 w146 w168 w182 w190 w221 _] -> w50
          tunnel: w49 -> [w71 w146 w168 w182 w190 w221 _]
          tunnel: [_ _ TRUE _ _ _ _] -> w48
          tunnel: w44 -> [w74 w145 w166 _ _ _ _]
          frame "False", Default {
            n272 = String Length(string=w71) -> (length=w69:i32)
            n273 = Greater?(x=w69, y=180) -> (0:w70:bool)
            n274 = local read "play"() -> (w76:bool)
            n275 = case shown="假" w70 {
              tunnel: [w128 ""] -> w105
              tunnel: w71 -> [w126 _]
              frame False {
                n276 = Format Date/Time String() -> (date/time string=w125:string)  [unwired: 3 in]
                "日期/时间" <- w125
                n277 = property on="State" class="Str"("Text.Scroll Position"=inf) -> ()  [unwired: 2 in, 2 out]
                n278 = Concatenate Strings(w126, "\n", w125, "通讯正常") -> (w128:string)
              }
              frame True {
              }
            }
            "State" <- w105
            n279 = case shown="真" w76 {
              frame False {
              }
              frame True {
                n280 = call "run _time_fgv .vi"() -> ("Value out"=w143:T15)  [unwired: 3 in, 1 out]
                n281 = call "Cycles_fgv.vi"() -> ("out"=→"CYC  Times":i32)  [unwired: 3 in, 1 out]
                n282 = Unbundle By Name(w143) -> ("time in"=→"Run Time":i32, "speed"=w140:dbl, "Torque"=w141:dbl)
                n283 = local write "设定Load[rpm]"(w140) -> ()
                n284 = local write "Set Torque[Nm]"(w141) -> ()
              }
            }
            n285 = case shown="真" w74 {
              tunnel: w123 -> [w133 w139]
              tunnel: [w133 w138] -> w121
              tunnel: [w134 w137] -> w114
              tunnel: w111 -> [w134 w135]
              tunnel: [w132 w136] -> w109
              frame False {
                w131 = 0.0 ("元素")
                n286 = Build Array(w131, w131, w131, w131, w131, w131, w131, w131) -> (w132:dbl[])
              }
              frame True {
                n287 = call "ykgw_read.vi"("error in (no error)"=w139, "Instrument in"=w135) -> ("error out"=w138:errorcluster, "Data out"=w136:dbl[], "Instrument out"=w137:refnum<class "Instrument.lvclass">)  [unwired: 7 in]
              }
            }
            n288 = Wait on Notification(notifier=w122, timeout in ms (-1)=500, error in (no error)=w121) -> (notification=w110:T16, timed out?=w116:bool, error out=w118:errorcluster)  [unwired: 1 in, 1 out]
            n289 = Equal?(x=w75, y="SaveData") -> (x = y?=w102:bool)
            n290 = Not(x=w116) -> (.not. x?=→"Torque":bool)
            n291 = call "gui_formatData.vi"("ykgw"=w109, "error in (no error)"=w118, "row size"=15, "Modbus Data"=w110, "Data in"=w119) -> ("error out"=w113:errorcluster, "report data"=w108:string[], "Data out"=w104:string[][], "SHOWN DATA"=w101:T17)  [unwired: 3 in]
            n292 = Unbundle By Name(w101) -> ("SHOWN"=w73:dbl[], "temp 1"=→"Temp 1":dbl, "temp 2"=→"Temp 2":dbl, "ECU EFF"=→"ECU EFF":dbl, "SYS EFF"=→"System EFF":dbl)
            n293 = Index Array(array=w73, index #1=0 ("索引"), index #2=1 ("索引"), index #3=2 ("索引"), index #4=3 ("索引"), index #5=4 ("索引"), index #6=5 ("索引"), index #7=6 ("索引"), index #8=7 ("索引"), index #9=8 ("索引"), index #10=9 ("索引")) -> (element #1=→"DC V":dbl, element #2=→"DCCurrent":dbl, element #3=→"DC Power":dbl, element #4=→"Pha V":dbl, element #5=→"Pha Current":dbl, element #6=→"Pha Power":dbl, element #7=→"Torque" →"Troque N/m":dbl, element #8=w77:dbl, element #9=→"Motor Power":dbl, element #10=→"Motor EFF":dbl)
            "r/m" <- w77
            n294 = Absolute Value(x=w77) -> (abs(x)=→"Speed":dbl)
            n295 = call "report_module.vi"("error in (no error)"=w113, "manual_save"=w102, "report_data"=w108, "Instrument in"=w114) -> ("error out"=w106:errorcluster, "Instrument out"=w107:refnum<class "Instrument.lvclass">)  [unwired: 6 in]
            n296 = call "Save Date.vi"("Save Data"=w104, "布尔"=w102) -> ("Save Data Out"=w103:string[][])  [unwired: 9 in]
            "DATA" <- w103
          }
          frame "Initialize" {
            w147 = string[][] [] ("Table Control")
            n297 = Variant To Data(error in=w159, type=refnum<class "Instrument.lvclass"> refnum ("Instrument.lvclass"), Variant=w158) -> (data=w156:refnum<class "Instrument.lvclass">, error out=w154:errorcluster)
            n298 = case shown="真" w145 {
              tunnel: w156 -> [w161 w165]
              tunnel: [w161 w164] -> w155
              tunnel: w154 -> [w160 w163]
              tunnel: [w160 w162] -> w153
              frame False {
              }
              frame True {
                n299 = call "ykgw_initialize.vi"("error in (no error)"=w163, "Instrument in"=w165) -> ("error out"=w162:errorcluster, "Instrument out"=w164:refnum<class "Instrument.lvclass">)  [unwired: 8 in]
              }
            }
            n300 = call "gui_formatTable.vi"() -> ("column size"=w148:u32, "column header"=w149:string[], "row size"=w150:u32, "row header"=w151:string[])  [unwired: 8 in]
            n301 = property on="DATA" class="Tbl (严格)"(error in=w153, "Row Headers[]"=w151, "Number of Rows"=w150, "Column Headers[]"=w149, "Number of Columns"=w148, "Value"=w147) -> (error out=w152:errorcluster)  [unwired: 1 in, 1 out]
          }
          frame "Shutdown" {
            n302 = call "report_close.vi"("error in (no error)"=w171, "Instrument in"=w169) -> ("error out"=w170:errorcluster, "Instrument out"=w172:refnum<class "Instrument.lvclass">)  [unwired: 8 in]
            n303 = case shown="真" w166 {
              tunnel: [w176 w181] -> w174
              tunnel: [w175 w180] -> w173
              tunnel: w172 -> [w176 w179]
              tunnel: w170 -> [w175 w178]
              frame False {
              }
              frame True {
                n304 = call "ykgw_close.vi"("error in (no error)"=w178, "DestroyAll"=TRUE, "Instrument in"=w179) -> ("error out"=w180:errorcluster, "Instrument out"=w181:refnum<class "Instrument.lvclass">)  [unwired: 7 in]
              }
            }
          }
          frame "CloseReport" {
            n305 = call "report_close.vi"("error in (no error)"=w189, "Instrument in"=w183) -> ("error out"=w186:errorcluster, "Instrument out"=w188:refnum<class "Instrument.lvclass">)  [unwired: 8 in]
            n306 = property on="Save data" class="Bool"(error in=w186, "Visible"=TRUE) -> (error out=w185:errorcluster)  [unwired: 1 in, 1 out]
          }
          frame "ConfigReport" {
            n307 = Variant To Data(error in=w206, type=T4 {"Path"=path "", "duration(min)"=0, "mode"=enum."Manual"} ("Cluster"), Variant=w205) -> (data=w199:T4, error out=w201:errorcluster)
            n308 = Unbundle By Name(w199) -> ("mode"=w198:T5)
            n309 = Equal?(x=core_reportMode."Manual", y=w198) -> (x = y?=w196:bool)
            n310 = Select(t="Save data" ("Boolean Text.Text"), s=w196, f="Stop") -> (s? t:f=w193:string)
            n311 = property on="Save data" class="Bool"(error in=w201, "BoolText.Text"=w193, "Visible"=TRUE) -> (error out=w200:errorcluster)  [unwired: 1 in, 1 out]
            n312 = call "report_config.vi"("error in (no error)"=w200, "Cluster"=w199, "Instrument in"=w191) -> ("error out"=w202:errorcluster, "Instrument out"=w203:refnum<class "Instrument.lvclass">)  [unwired: 7 in]
          }
          frame "StopAuto" {
            w210 = T18."Enabled" ("禁用")
            w211 = FALSE ("值(信号)")
            n313 = local read "Speed"() -> (w219:dbl)
            n314 = Unbundle By Name(w225) -> ("modbus"=w224:T11, "ecu"=w223:T11)
            n315 = Greater?(x=w219, y=100.0) -> (0:w218:bool)
            n316 = case shown="真" w218 {
              tunnel: w224 -> [w231 w244]
              tunnel: w223 -> [w232 w243]
              tunnel: w222 -> [_ w241]
              tunnel: [w228 w239] -> w216
              tunnel: [w229 w240] -> w217
              frame False {
                w233 = 0 ("设定Load[rpm]")
                w230 = 0.0
                n317 = local write "Set LoadDivide"(w230) -> ()
                n318 = Bundle By Name(cluster=T12 {"cmd"="SetTorque", "data"=variant} ("element"), "data"=w230) -> (w236:T12)
                n319 = Bundle By Name(cluster=T12 {"cmd"="SetSpeed", "data"=variant} ("element"), "data"=w233) -> (w238:T12)
                n320 = local write "设定Load[rpm]"(w233) -> ()
                n321 = Enqueue Element(queue=w232, element=w236) -> (error out=w237:errorcluster)  [unwired: 2 in, 2 out]
                n322 = Enqueue Element(queue=w231, element=w238, error in (no error)=w237) -> (error out=w228:errorcluster)  [unwired: 1 in, 2 out]
                n323 = Get Date/Time In Seconds() -> (seconds since 1Jan1904=w229:timestamp)
              }
              frame True {
                n324 = for {
                  N: 10 -> [_]
                  tunnel: w241 -> [w259]
                  tunnel: w244 -> [w255]
                  tunnel: w243 -> [w251]
                  tunnel: [w246] -> w240
                  tunnel: [w245] -> w239
                  i -> [w254]
                  stop <- w257 stop-if-true
                  n325 = Wait (ms)(milliseconds to wait=u32 600 ("等待时间（毫秒）")) -> ()  [unwired: 1 out]
                  n326 = Greater?(x=w254, y=6) -> (0:w252:bool)
                  n327 = Greater?(x=w254, y=8) -> (0:w257:bool)
                  n328 = case shown="真" w252 {
                    tunnel: [100 ("设定Load[rpm]") 0 ("设定Load[rpm]")] -> w249
                    tunnel: [1.0 0.0] -> w248
                    frame False {
                    }
                    frame True {
                    }
                  }
                  n329 = local write "Set Torque[Nm]"(w248) -> ()
                  n330 = Bundle By Name(cluster=T12 {"cmd"="SetTorque", "data"=variant} ("element"), "data"=w248) -> (w261:T12)
                  n331 = local write "设定Load[rpm]"(w249) -> ()
                  n332 = Enqueue Element(queue=w251, element=w261, error in (no error)=w259) -> (error out=w260:errorcluster)  [unwired: 1 in, 2 out]
                  n333 = Get Date/Time In Seconds() -> (seconds since 1Jan1904=w246:timestamp)
                  n334 = Bundle By Name(cluster=T12 {"cmd"="SetSpeed", "data"=variant} ("element"), "data"=w249) -> (w262:T12)
                  n335 = Enqueue Element(queue=w255, element=w262, error in (no error)=w260) -> (error out=w245:errorcluster)  [unwired: 1 in, 2 out]
                }
              }
            }
            "Finish Time" <- w217
            n336 = property on="play" class="Bool (严格)"(error in=w216, "Val(Sgnl)"=w211) -> (error out=w215:errorcluster)  [unwired: 1 in, 1 out]
            n337 = property on="emergency stop" class="Bool (严格)"(error in=w215, "Val(Sgnl)"=w211) -> (error out=w214:errorcluster)  [unwired: 1 in, 1 out]
            n338 = property on="ECU ACK" class="Bool"(error in=w214, "DisabledEnum"=w210) -> (error out=w213:errorcluster)  [unwired: 1 in, 1 out]
            n339 = property on="LOAD ACK" class="Bool"(error in=w213, "DisabledEnum"=w210) -> (error out=w212:errorcluster)  [unwired: 1 in, 1 out]
            n340 = property on="ecu" class="Bool (严格)"(error in=w212, "DisabledEnum"=w210) -> (error out=w209:errorcluster)  [unwired: 1 in, 1 out]
            n341 = property on="load 2" class="Bool (严格)"(error in=w209, "DisabledEnum"=w210) -> (error out=w208:errorcluster)  [unwired: 1 in, 1 out]
          }
          frame "emergency stop" {
            n342 = Unbundle By Name(w271) -> ("modbus"=w270:T11, "ecu"=w269:T11)
            n343 = for {
              N: 35 -> [_]
              tunnel: w270 -> [w288]
              tunnel: w269 -> [w285]
              tunnel: [w278] -> w267
              i -> [w287]
              stop <- w276 stop-if-true
              n344 = local read "Speed"() -> (w274:dbl)
              n345 = Wait (ms)(milliseconds to wait=u32 600 ("等待时间（毫秒）")) -> ()  [unwired: 1 out]
              n346 = Greater?(x=w287, y=5) -> (0:w280:bool)
              n347 = Greater?(x=w287, y=33) -> (0:w277:bool)
              n348 = Less?(x=w274, y=100.0) -> (x < y?=w279:bool)
              n349 = Or(x=w279, y=w280) -> (x .or. y?=w281:bool)
              n350 = case shown="真" w281 {
                tunnel: [100 ("设定Load[rpm]") 0 ("设定Load[rpm]")] -> w272
                tunnel: [2.0 0.0] -> w273
                tunnel: [FALSE TRUE] -> w275
                frame False {
                }
                frame True {
                }
              }
              n351 = Or(x=w275, y=w277) -> (x .or. y?=w276:bool)
              n352 = Bundle By Name(cluster=T12 {"cmd"="SetTorque", "data"=variant} ("element"), "data"=w273) -> (w292:T12)
              n353 = local write "设定Load[rpm]"(w272) -> ()
              n354 = Enqueue Element(queue=w285, element=w292) -> (error out=w291:errorcluster)  [unwired: 2 in, 2 out]
              n355 = Bundle By Name(cluster=T12 {"cmd"="SetSpeed", "data"=variant} ("element"), "data"=w272) -> (w293:T12)
              n356 = Enqueue Element(queue=w288, element=w293, error in (no error)=w291) -> (error out=w278:errorcluster)  [unwired: 1 in, 2 out]
            }
          }
        }
        n357 = disable-structure shown="启用" {
          disable-tunnel: [w65 w66] -> w57
          disable-tunnel: w43 -> [w64 w67]
          frame Disabled {
            n358 = call "Error_Handler.vi"("error in"=w64) -> ("error out"=w65:errorcluster)  [unwired: 8 in, 2 out]
          }
          frame Enabled {
            n359 = call <vilib>:"Clear Errors.vi"("error in (no error)"=w67) -> ("error out"=w66:errorcluster)  [unwired: 5 in, 1 out]
          }
        }
      }
    }
    frame Error {
    }
  }
  n360 = Merge Errors(w18, w20, w22, w17) -> (w21:errorcluster)
  n361 = call "core_module.vi"("error in (no error)"=w21) -> ("error out"=w7:errorcluster)  [unwired: 6 in, 4 out]
  n362 = disable-structure shown="RUN_TIME_ENGINE==True" {
    disable-tunnel: w7 -> [_ _]
    frame condition #0 (active) {
    }
    frame condition #1 {
      n363 = Quit LabVIEW() -> ()  [unwired: 1 in]
    }
  }
